vi "Get_Indexes_and_Number_of_Jumps(Other_Origin)-5.vi"(4 "[IN] Minimal Subtrack\nLength for Making Desicion":i32, 5 "[IN] Indexes for Jumps\nfrom Previous Origin":i32[](array[numeric]), 7 "error IN":errorcluster, 8 "[IN] # of Track with\nFirst Problem Point":i32, 9 "[IN] Index of First Pro\nblem Point Inside Track":i32, 10 "[IN] Still connected\ntracks in group":T1) -> (0 "error OUT":errorcluster, 2 "[OUT] # of case":u8, 3 "[OUT] Indexes for Jumps\nFROM new Origin":i32[](array[numeric]))   [LabVIEW 2013]
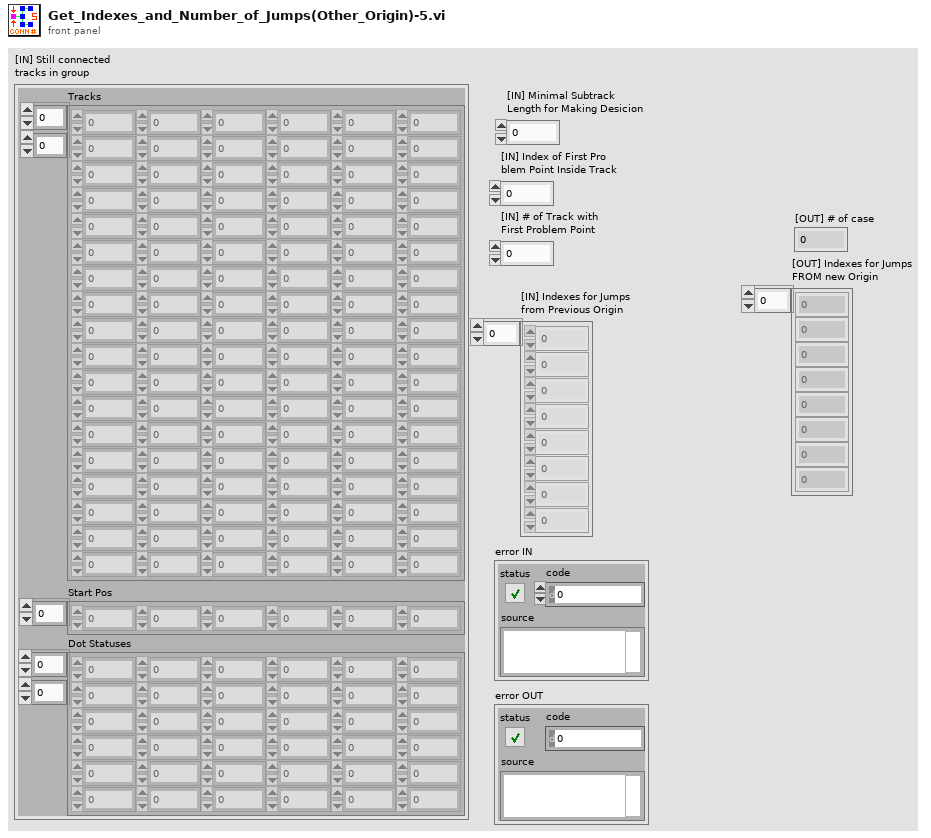
[diagram p1: front panel]
types:
  T1 = cluster{"Tracks":dbl[][], "Start Pos":i32[], "Dot Statuses":i16[][]}
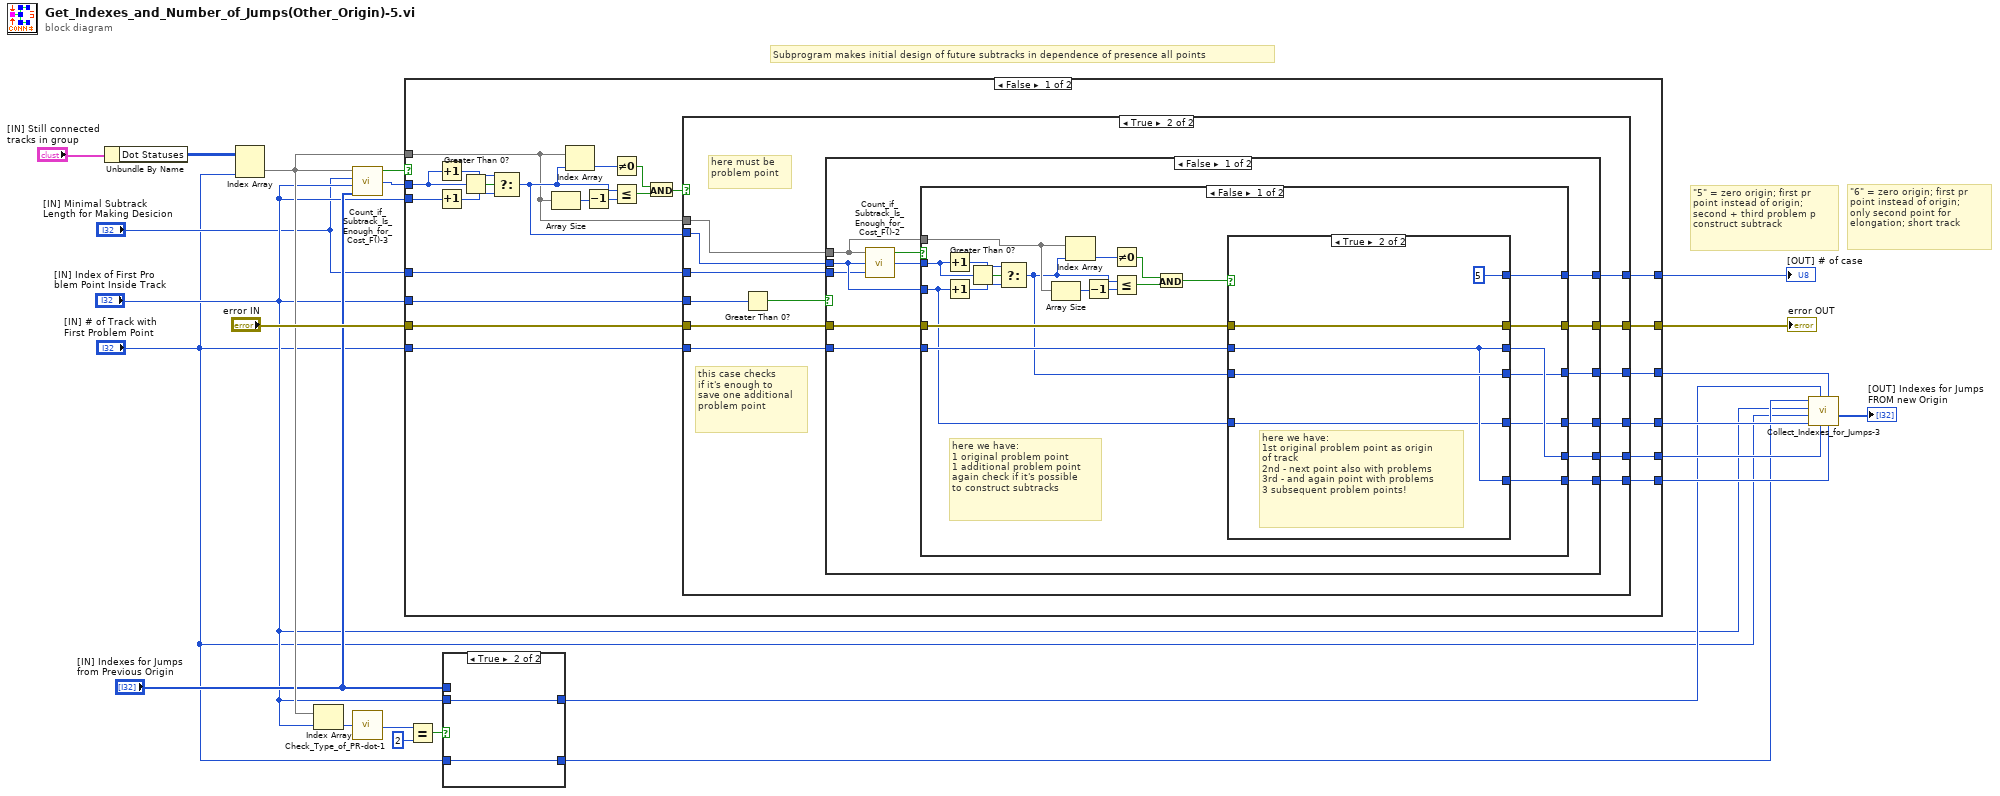
[diagram p0: block diagram]
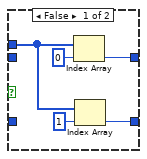
[diagram p2: hidden frame]
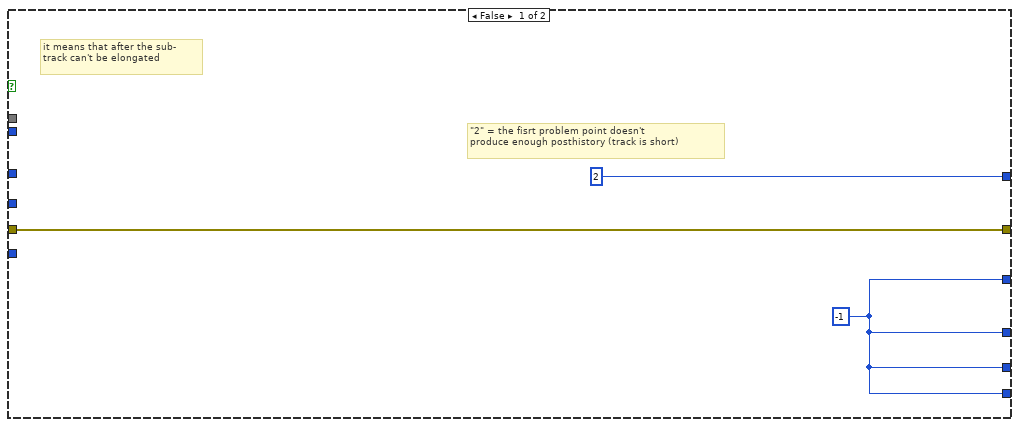
[diagram p3: hidden frame]
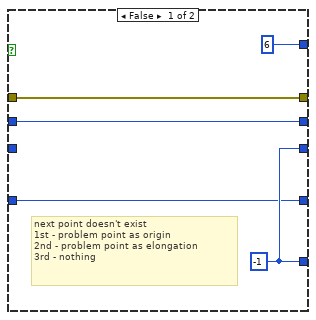
[diagram p4: hidden frame]
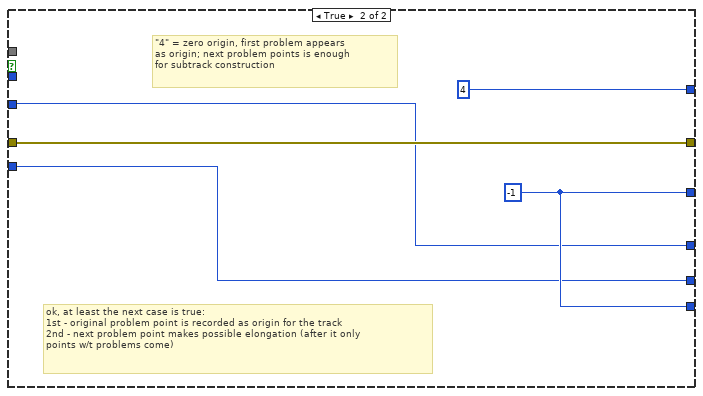
[diagram p5: hidden frame]
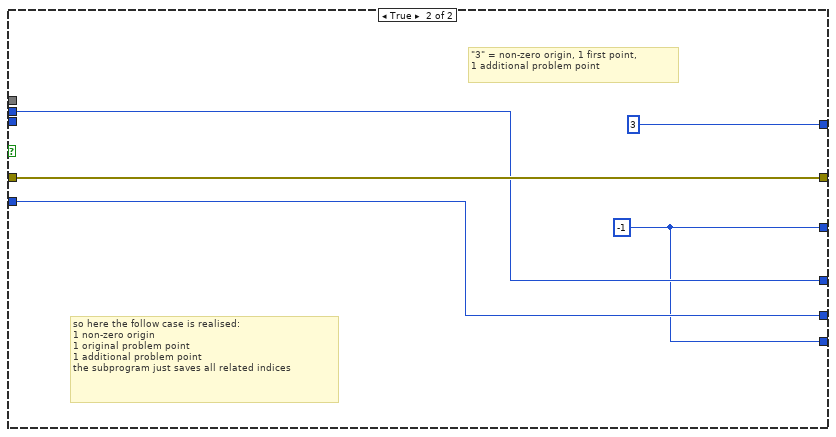
[diagram p6: hidden frame]
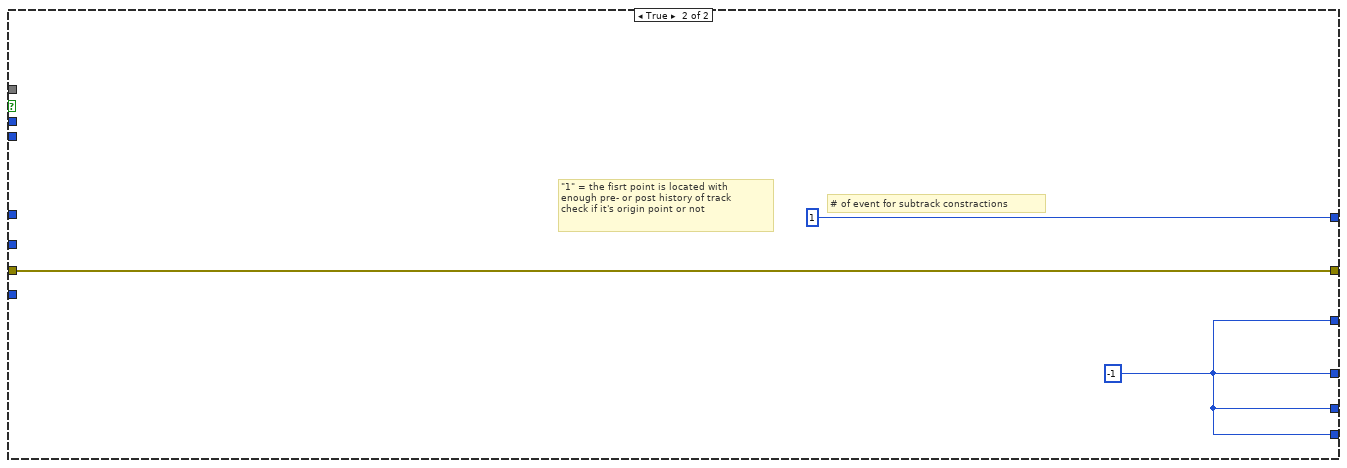
[diagram p7: hidden frame]
diagram:
  # "\"6\" = zero origin; first pr \npoint instead of origin; \nonly second point for \nelongation; short track"
  # "\"5\" = zero origin; first pr \npoint instead of origin; \nsecond + third problem p\nconstruct subtrack"
  # "Subprogram makes initial design of future subtracks in dependence of presence all points"
  n1 = Unbundle By Name("[IN] Still connected\ntracks in group") -> ("Dot Statuses"=w22:i16[][])
  n2 = Index Array(array=w22, index (col)="[IN] # of Track with\nFirst Problem Point") -> (element=w7:i16[])  [unwired: 1 in]
  n3 = Index Array(array=w7, index="[IN] Index of First Pro\nblem Point Inside Track") -> (element=w18:i16)
  n4 = call "Count_if_Subtrack_Is_Enough_for_Cost_F()-3.vi"("[IN] Indexes for Jumps\nfrom Previous Origin"="[IN] Indexes for Jumps\nfrom Previous Origin", "[IN] Index of Problem \nPoint Inside Track"="[IN] Index of First Pro\nblem Point Inside Track", "[IN] Minimal Subtrack Length \n(Points without problems) for\nMaking Desicion"="[IN] Minimal Subtrack\nLength for Making Desicion", "[IN] Dot Statuses in Track"=w7) -> ("[OUT] Index of Last \nPoint in Track"=w5:i32, "[OUT] It's enough to make\nconclusion using subtrack"=w6:bool)  [unwired: 1 in]
  n5 = call "Check_Type_of_PR-dot-1.vi"("[IN] dot status"=w18) -> ("[OUT] Type of\nproblem dot"=w17:i32)
  n6 = case shown="False" w6 {
    tunnel: w5 -> [w44 _]
    tunnel: "[IN] Index of First Pro\nblem Point Inside Track" -> [w42 _]
    tunnel: w7 -> [w32 _]
    tunnel: "[IN] Index of First Pro\nblem Point Inside Track" -> [w34 _]
    tunnel: "[IN] # of Track with\nFirst Problem Point" -> [w33 _]
    tunnel: "[IN] Minimal Subtrack\nLength for Making Desicion" -> [w31 _]
    tunnel: "error IN" -> [w30 w119]
    tunnel: [w29 w119] -> w20
    tunnel: [w28 u8 1] -> w19
    tunnel: [w26 w117] -> w14
    tunnel: [w25 w117] -> w13
    tunnel: [w27 w117] -> w12
    tunnel: [w24 w117] -> w11
    frame False {
      n7 = Increment(x=w44) -> (x+1=w45:i32)
      n8 = Increment(x=w42) -> (x+1=w43:i32)
      n9 = Greater Than 0?(x=w44) -> (x > 0?=w46:bool)
      n10 = Select(t=w45, s=w46, f=w43) -> (s? t:f=w35:i32)
      n11 = Array Size(array=w32) -> (size(s)=w41:i32)
      n12 = Index Array(array=w32, index=w35) -> (element=w38:i16)
      n13 = Decrement(x=w41) -> (x-1=w40:i32)
      n14 = Not Equal To 0?(x=w38) -> (x != 0?=w37:bool)
      n15 = Less Or Equal?(x=w35, y=w40) -> (x <= y?=w39:bool)
      n16 = And(x=w37, y=w39) -> (x .and. y?=w36:bool)
      n17 = case shown="True" w36 {
        tunnel: w35 -> [_ w59]
        tunnel: w34 -> [_ w58]
        tunnel: w33 -> [_ w62]
        tunnel: w32 -> [_ w61]
        tunnel: w31 -> [_ w60]
        tunnel: w30 -> [w49 w56]
        tunnel: [w49 w55] -> w29
        tunnel: [u8 2 w54] -> w28
        tunnel: [w47 w51] -> w27
        tunnel: [w47 w53] -> w26
        tunnel: [w47 w52] -> w25
        tunnel: [w47 w50] -> w24
        frame False {
          w47 = -1
          # "\"2\" = the fisrt problem point doesn't \nproduce enough posthistory (track is short)"
          # "it means that after the sub-\ntrack can't be elongated"
        }
        frame True {
          # "this case checks\nif it's enough to\nsave one additional\nproblem point"
          # "here must be \nproblem point"
          n18 = Greater Than 0?(x=w58) -> (x > 0?=w57:bool)
          n19 = case shown="False" w57 {
            tunnel: w62 -> [w73 w113]
            tunnel: w61 -> [w67 _]
            tunnel: w60 -> [w65 _]
            tunnel: w59 -> [w66 w114]
            tunnel: w56 -> [w75 w116]
            tunnel: [w74 w116] -> w55
            tunnel: [w72 u8 3] -> w54
            tunnel: [w69 w114] -> w53
            tunnel: [w68 w113] -> w52
            tunnel: [w71 w112] -> w51
            tunnel: [w70 w112] -> w50
            frame False {
              n20 = call "Count_if_Subtrack_Is_Enough_for_Cost_F()-2.vi"("[IN] Minimal Subtrack Length \n(Points without problems) for\nMaking Desicion"=w65, "[IN] Index of Problem \nPoint Inside Track"=w66, "[IN] Dot Statuses in Track"=w67) -> ("[OUT] Index of Last \nPoint in Track"=w64:i32, "[OUT] It's enough to make\nconclusion using subtrack"=w63:bool)  [unwired: 1 in]
              n21 = case shown="False" w63 {
                tunnel: w64 -> [w93 _]
                tunnel: w66 -> [w77 w107]
                tunnel: w67 -> [w87 _]
                tunnel: w75 -> [w86 w111]
                tunnel: [w85 w111] -> w74
                tunnel: w73 -> [w84 w108]
                tunnel: [w82 u8 4] -> w72
                tunnel: [w80 w109] -> w71
                tunnel: [w79 w109] -> w70
                tunnel: [w78 w107] -> w69
                tunnel: [w81 w108] -> w68
                frame False {
                  # "here we have:\n1 original problem point\n1 additional problem point\nagain check if it's possible \nto construct subtracks"
                  n22 = Increment(x=w93) -> (x+1=w95:i32)
                  n23 = Increment(x=w77) -> (x+1=w94:i32)
                  n24 = Greater Than 0?(x=w93) -> (x > 0?=w96:bool)
                  n25 = Select(t=w95, s=w96, f=w94) -> (s? t:f=w83:i32)
                  n26 = Array Size(array=w87) -> (size(s)=w92:i32)
                  n27 = Index Array(array=w87, index=w83) -> (element=w89:i16)
                  n28 = Decrement(x=w92) -> (x-1=w91:i32)
                  n29 = Not Equal To 0?(x=w89) -> (x != 0?=w88:bool)
                  n30 = Less Or Equal?(x=w83, y=w91) -> (x <= y?=w90:bool)
                  n31 = And(x=w88, y=w90) -> (x .and. y?=w76:bool)
                  n32 = case shown="True" w76 {
                    tunnel: [w101 w106] -> w85
                    tunnel: w86 -> [w101 w106]
                    tunnel: w84 -> [w99 w103]
                    tunnel: w83 -> [_ w104]
                    tunnel: [u8 6 u8 5] -> w82
                    tunnel: [w99 w103] -> w81
                    tunnel: [w98 w104] -> w80
                    tunnel: [w98 w103] -> w79
                    tunnel: [w97 w102] -> w78
                    tunnel: w77 -> [w97 w102]
                    frame False {
                      w98 = -1 ("[IN] # of Track with\nFirst Problem Point")
                      # "next point doesn't exist\n1st - problem point as origin\n2nd - problem point as elongation\n3rd - nothing"
                    }
                    frame True {
                      # "here we have:\n1st original problem point as origin\nof track\n2nd - next point also with problems\n3rd - and again point with problems\n3 subsequent problem points!"
                    }
                  }
                }
                frame True {
                  w109 = -1
                  # "\"4\" = zero origin, first problem appears\nas origin; next problem points is enough \nfor subtrack construction"
                  # "ok, at least the next case is true: \n1st - original problem point is recorded as origin for the track\n2nd - next problem point makes possible elongation (after it only \npoints w/t problems come)"
                }
              }
            }
            frame True {
              w112 = -1
              # "\"3\" = non-zero origin, 1 first point, \n1 additional problem point"
              # "so here the follow case is realised:\n1 non-zero origin \n1 original problem point\n1 additional problem point\nthe subprogram just saves all related indices"
            }
          }
        }
      }
    }
    frame True {
      w117 = -1
      # "\"1\" = the fisrt point is located with \nenough pre- or post history of track\ncheck if it's origin point or not"
      # "# of event for subtrack constractions"
    }
  }
  "error OUT" <- w20
  "[OUT] # of case" <- w19
  n33 = Equal?(x=w17, y=2) -> (x = y?=w15:bool)
  n34 = case shown="True" w15 {
    tunnel: [w123 w125] -> w8
    tunnel: "[IN] Index of First Pro\nblem Point Inside Track" -> [_ w125]
    tunnel: [w121 w126] -> w9
    tunnel: "[IN] # of Track with\nFirst Problem Point" -> [_ w126]
    tunnel: "[IN] Indexes for Jumps\nfrom Previous Origin" -> [w120 _]
    frame False {
      n35 = Index Array(array=w120, index=0) -> (element=w123:i32)
      n36 = Index Array(array=w120, index=1) -> (element=w121:i32)
    }
    frame True {
    }
  }
  n37 = call "Collect_Indexes_for_Jumps-3.vi"("[IN] # Track with \nThird Problem Point"=w11, "[IN] Index of Third\nProblem point"=w12, "[IN] # Track with \nSecond Problem Point"=w13, "[IN] Index of Point Be\nfore Problem (Origin)"=w8, "[IN] Index of Second\nProblem point"=w14, "[IN] # Track with First\nProblem Point"="[IN] # of Track with\nFirst Problem Point", "[IN] Index of First \nProblem Point"="[IN] Index of First Pro\nblem Point Inside Track", "[IN] # Track of Origin"=w9) -> ("[OUT] Indexes for Jumps"=→"[OUT] Indexes for Jumps\nFROM new Origin":i32[])  [unwired: 3 in]
